vi "Error PLC.vi"(8 "error in":errorcluster, 11 "String":string) -> (0 "error out":errorcluster)   [LabVIEW 2015, in "PLC.lvlib"]
uses:
  PLC.lvlib
  support/Message Queue/Message Queue.lvlib
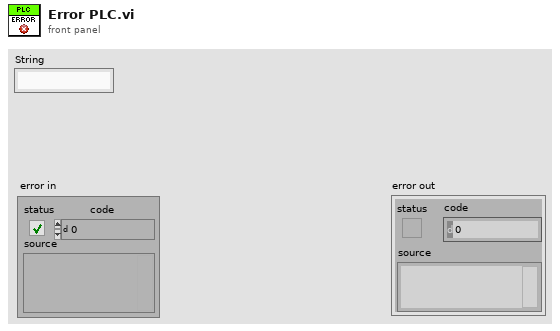
[diagram p1: front panel]
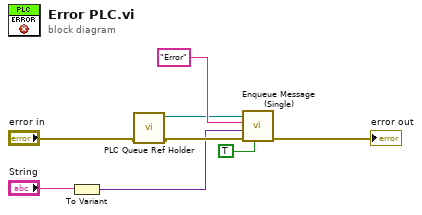
[diagram p0: block diagram]
diagram:
  n1 = To Variant(anything="String") -> (Variant=w3:variant)
  n2 = call "PLC Queue Ref Holder.vi"("error in"="error in") -> ("error out"=w4:errorcluster, "Input Message Queue"=w5:refnum<queue>)  [unwired: 9 in]
  n3 = call "Enqueue Message (Single).vi"("Priority Message? (F)"=TRUE, "error in (no error)"=w4, "Message Data"=w3, "Message"="Error", "Message Queue"=w5) -> ("error out"=→"error out":errorcluster)  [unwired: 5 in, 1 out]
